vi "test enumerate.vi"() -> ()   [LabVIEW 2013, in "TBM Tests.lvlib"]
uses:
  TBM Tests.lvlib
  root configuration/TBM configuration.lvclass
panel:
  out "subtreeok":bool
  out "subok":bool
  out "data ok":bool
  out "topok":bool
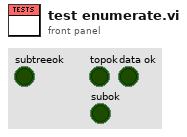
[diagram p1: front panel]
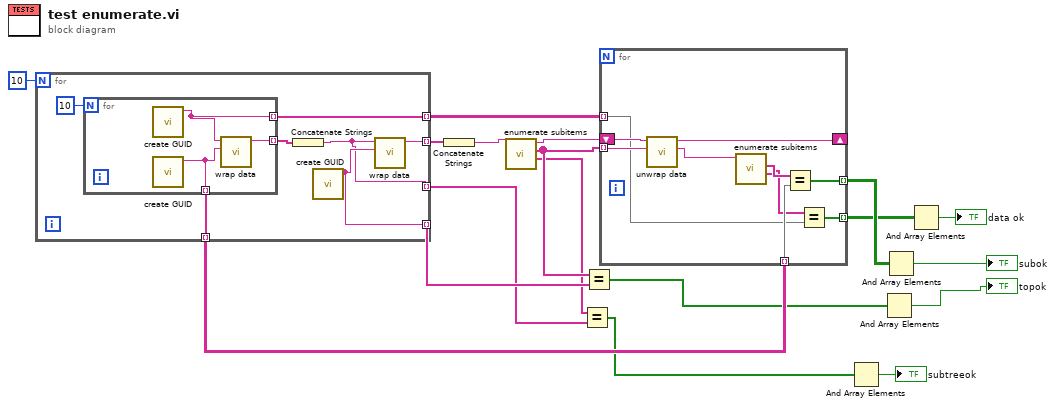
[diagram p0: block diagram]
diagram:
  n1 = for {
    N: 10 -> [_]
    tunnel: [w23] -> w17 mode=indexing
    tunnel: [w22] -> w15 mode=indexing
    tunnel: [w21] -> w12 mode=indexing
    tunnel: [w20] -> w8 mode=indexing
    tunnel: [w19] -> w3 mode=indexing
    n2 = for {
      N: 10 -> [_]
      tunnel: [w28] -> w24 mode=indexing
      tunnel: [w27] -> w21 mode=indexing
      tunnel: [w26] -> w20 mode=indexing
      n3 = call "create GUID.vi"() -> ("uuid"=w26:string)  [unwired: 11 in]
      n4 = call "create GUID.vi"() -> ("uuid"=w27:string)  [unwired: 11 in]
      n5 = call "wrap data.vi"("identifier"=w27, "data to wrap"=w26) -> ("wrapped data"=w28:string)  [unwired: 9 in]
    }
    n6 = Concatenate Strings(w24) -> (w19:string)
    n7 = call "create GUID.vi"() -> ("uuid"=w22:string)  [unwired: 11 in]
    n8 = call "wrap data.vi"("identifier"=w22, "data to wrap"=w19) -> ("wrapped data"=w23:string)  [unwired: 9 in]
  }
  n9 = Concatenate Strings(w17) -> (w16:string)
  n10 = call "enumerate subitems.vi"("data to enumerate"=w16) -> ("associated data"=w4:string[], "discovered subitems"=w14:string[], "data out"=w13:string)  [unwired: 8 in]
  n11 = Equal?(x=w4, y=w3) -> (x = y?=w2:bool[])
  n12 = Equal?(x=w14, y=w15) -> (x = y?=w10:bool[])
  n13 = for {
    tunnel: w14 -> [w36] mode=indexing
    shift-right: [w37] -> _
    shift-left: w13 -> [w38]
    tunnel: w12 -> [w33] mode=indexing
    tunnel: [w32] -> w11 mode=indexing
    tunnel: w8 -> [w30] mode=indexing
    tunnel: [w29] -> w7 mode=indexing
    n14 = call "unwrap data.vi"("identifier"=w36, "data to unwrap"=w38) -> ("unwrapped data"=w35:string, "remaining string"=w37:string)  [unwired: 8 in]
    n15 = call "enumerate subitems.vi"("data to enumerate"=w35) -> ("associated data"=w31:string[], "discovered subitems"=w34:string[])  [unwired: 8 in, 1 out]
    n16 = Equal?(x=w34, y=w33) -> (x = y?=w32:bool[])
    n17 = Equal?(x=w31, y=w30) -> (x = y?=w29:bool[])
  }
  n18 = And Array Elements(Boolean array=w2) -> (logical AND=→"subtreeok":bool)
  n19 = And Array Elements(Boolean array=w10) -> (logical AND=→"topok":bool)
  n20 = And Array Elements(Boolean array=w11) -> (logical AND=→"subok":bool)
  n21 = And Array Elements(Boolean array=w7) -> (logical AND=→"data ok":bool)
